vi "Get error type.vi"(8 "error in":errorcluster, 10 "error to look up":errorcluster) -> (0 "error out":errorcluster, 1 "Station and step":string, 2 "Description":string, 3 "Error Type":T1)   [LabVIEW 2018, in "Error Handler.lvlib"]
uses:
  Error Handler.lvlib
  ctl/Error Type.ctl
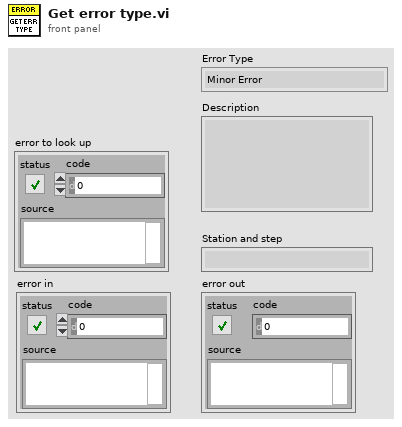
[diagram p1: front panel]
types:
  T1 = typedef "Error Handler.lvlib/Error Type.ctl" = enum16{"Minor Error", "Wash Cycle Error", "System Error"}
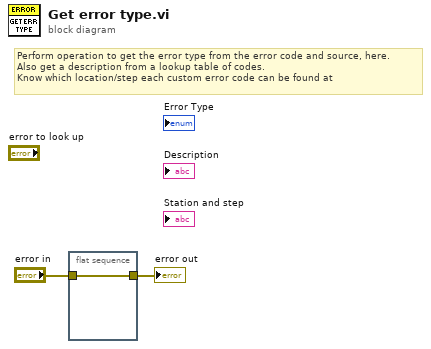
[diagram p0: block diagram]
diagram:
  # "Perform operation to get the error type from the error code and source, here.\nAlso get a description from a lookup table of codes.\nKnow which location/step each custom error code can be found at"
  n1 = flat-sequence {
    tunnel: "error in" -> [w3]
    tunnel: [w3] -> w1
    frame #0 {
    }
  }
  "error out" <- w1
